vi "synnax writer commit.vi"(8 "error in":errorcluster, 11 "Writer":refnum<class "Synnax Writer.lvclass">) -> (0 "error out":errorcluster, 2 "out_end_ts":i64, 3 "Writer Out":refnum<class "Synnax Writer.lvclass">)   [LabVIEW 2026, in "synnax_clib.lvlib" / "Synnax Writer.lvclass"]
doc: "synnax_writer_commit(SynnaxWriter writer, int64_t *out_end_ts, SynnaxError err);"
uses:
  Synnax Writer.lvclass
  Synnax Writer.lvclass/Synnax Writer.ctl
  synnax_clib.dll
  synnax_clib.lvlib
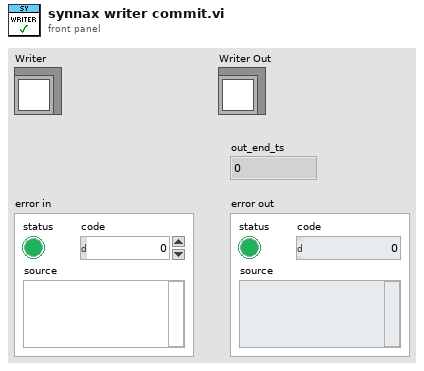
[diagram p1: front panel]
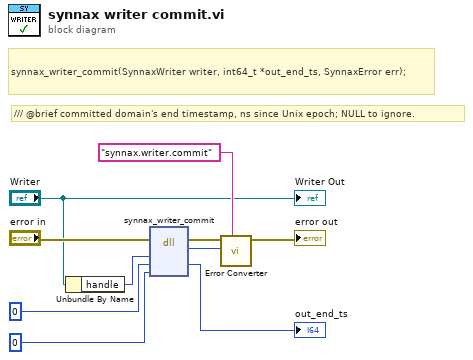
[diagram p0: block diagram]
diagram:
  # "/// @brief committed domain's end timestamp, ns since Unix epoch; NULL to ignore."
  # "synnax_writer_commit(SynnaxWriter writer, int64_t *out_end_ts, SynnaxError err);"
  n1 = Unbundle By Name("Writer") -> ("handle"=w1:u64)
  n2 = dll-call lib="C/synnax/client/labview/synnax_clib.*" fn="synnax_writer_commit"(error in="error in", "writer"=w1, "out_end_ts"=i64 0, "err"=u64 0) -> (error out=w7:errorcluster, w6:i32, "out_end_ts"=→"out_end_ts":i64)  [unwired: 4 in, 1 out]
  n3 = call "Error Converter.vi"("source"="synnax.writer.commit", "error code"=w6, "error in (no error)"=w7) -> ("error out"=→"error out":errorcluster)  [unwired: 8 in]
  "Writer Out" <- "Writer"
